vi "Pololu.Mgr - Store Lower or Upper Stop Position.vi"(6 "Type":enum16{"Lower", "Upper"}(ring), 8 "error in (no error)":errorcluster, 9 "Pos(Deg)":dbl, 10 "Channel":u8, 11 "PololuCtrl in":refnum<class "PololuCtrl.lvclass">) -> (0 "error out":errorcluster, 2 "Device Config":T1[](array[typedef]), 3 "PololuCtrl out":refnum<class "PololuCtrl.lvclass">)   [LabVIEW 2018, in "PololuCtrl.lvclass"]
uses:
  PololuCtrl.lvclass
  SubVIs/Pololu.Device Config.ctl
  SubVIs/Pololu.Device Range Config.ctl
  PololuCtrl.lvclass/PololuCtrl.ctl
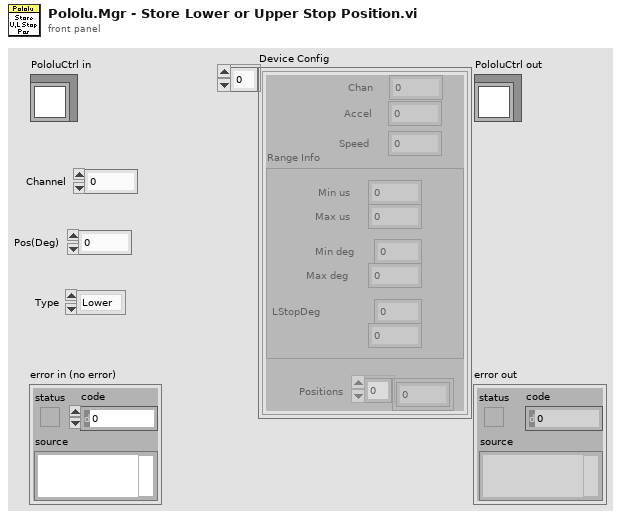
[diagram p1: front panel]
types:
  T1 = typedef "Pololu.Device Config.ctl" = cluster{"Chan":u8, "Accel":u16, "Speed":u16, "Positions":dbl[], "Range Info":T2}
  T2 = typedef "Pololu.Device Range Config.ctl" = cluster{"Min us":dbl, "Max us":dbl, "Min deg":dbl, "Max deg":dbl, "LStopDeg":dbl, "UStopDeg":dbl}
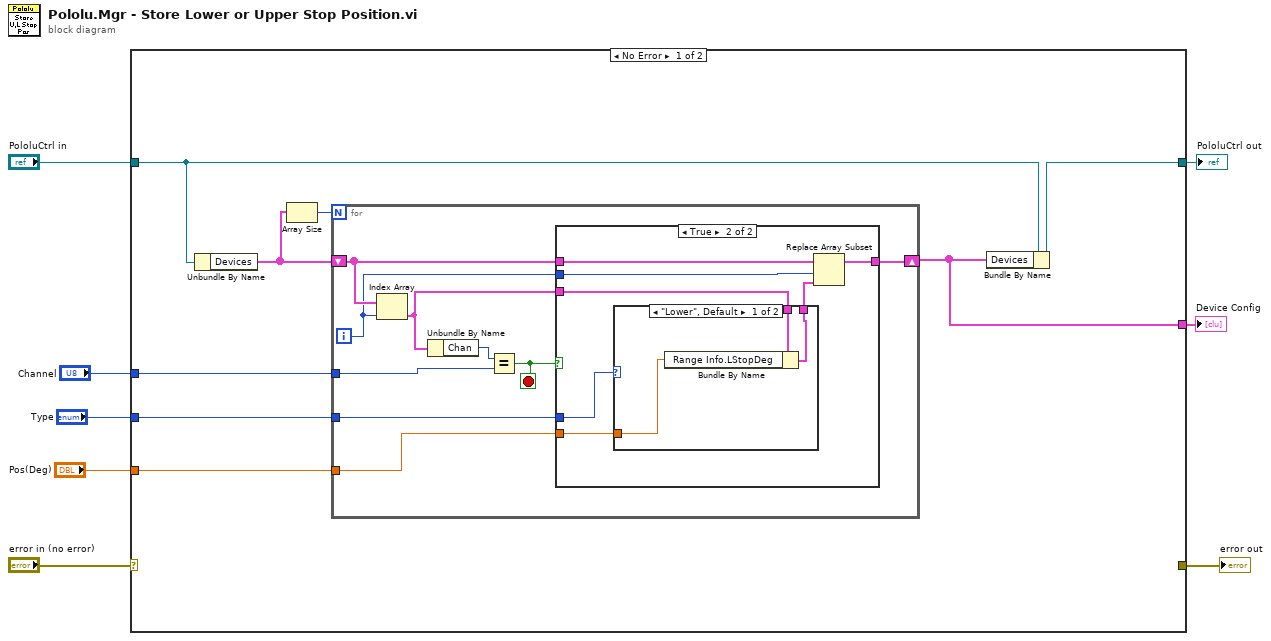
[diagram p0: block diagram]
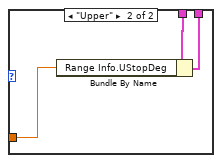
[diagram p3: hidden frame]
diagram:
  n1 = case shown="No Error" "error in (no error)" {
    selector: "error in (no error)" -> [_ w41]
    tunnel: [_ w41] -> w7
    tunnel: [w14 w40] -> w5
    tunnel: "PololuCtrl in" -> [w15 w40]
    tunnel: "Channel" -> [w16 _]
    tunnel: "Pos(Deg)" -> [w11 _]
    tunnel: [w13 _] -> w2
    tunnel: "Type" -> [w12 _]
    frame No Error {
      n2 = Unbundle By Name(w15) -> ("Devices"=w10:T1[])
      n3 = Array Size(array=w10) -> (size(s)=w9:i32)
      n4 = for {
        N: w9 -> [_]
        shift-right: [w21] -> w13
        shift-left: w10 -> [w22]
        tunnel: w16 -> [w24]
        tunnel: w12 -> [w18]
        tunnel: w11 -> [w17]
        i -> [w20]
        stop <- w23 stop-if-true
        n5 = Index Array(array=w22, index=w20) -> (element=w19:T1)
        n6 = Unbundle By Name(w19) -> ("Chan"=w25:u8)
        n7 = Equal?(x=w25, y=w24) -> (x = y?=w23:bool)
        n8 = case shown="True" w23 {
          tunnel: w22 -> [w26 w33]
          tunnel: [w26 w32] -> w21
          tunnel: w20 -> [_ w31]
          tunnel: w19 -> [_ w30]
          tunnel: w18 -> [_ w28]
          tunnel: w17 -> [_ w27]
          frame False {
          }
          frame True {
            n9 = case shown="\"Lower\", Default" w28 {
              tunnel: w30 -> [w36 w39]
              tunnel: [w35 w38] -> w29
              tunnel: w27 -> [w34 w37]
              frame "Lower", Default {
                n10 = Bundle By Name(cluster=w36, "Range Info.LStopDeg"=w34) -> (w35:T1)
              }
              frame "Upper" {
                n11 = Bundle By Name(cluster=w39, "Range Info.UStopDeg"=w37) -> (w38:T1)
              }
            }
            n12 = Replace Array Subset(array=w33, new element=w29, index=w31) -> (w32:T1[])
          }
        }
      }
      n13 = Bundle By Name(cluster=w15, "Devices"=w13) -> (w14:refnum<class "PololuCtrl.lvclass">)
    }
    frame Error {
    }
  }
  "error out" <- w7
  "PololuCtrl out" <- w5
  "Device Config" <- w2
